vi "Extract Doubles.vi"(1 "String":string="53k, 42M, 37u", 2 "Eng Units?":bool) -> (0 "Data":dbl[](array[numeric]) format="%.5e")   [LabVIEW 2018]
doc: "Finds all numbers in the given string and puts them into an array as double-precision numbers. All of the following formats are recognized:\n123 1.23 1.23e2 1.23E2\nNo spaces or other characters may appear within the number, but any characters may appear before or after the number.\nThe engineering units convers suffixes k,m,u as 1000, 0.001 and 1e-6 multipliers. Case of the units is not important which means that \"M\" is the same as \"m\" and denotes a 0.001 multiplier.\nModified from examples which did not work, by\nScott Hannahs, <sth@magnet.fsu.edu> NHMFL-FSU, May 2003\nAuthor: Scott Hannahs <sth@magnet.fsu.edu>\nCopyright 2018 Florida State University, All rights reserved."
panel:
  # "This VI takes a string containing multiple numbers and\nextracts those numbers into an array.  See the Get Info\ndialog box for more information."
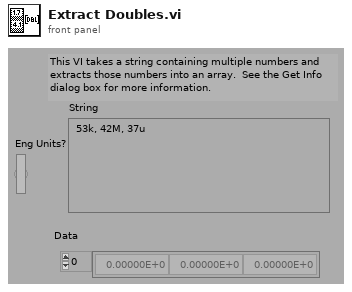
[diagram p1: front panel]
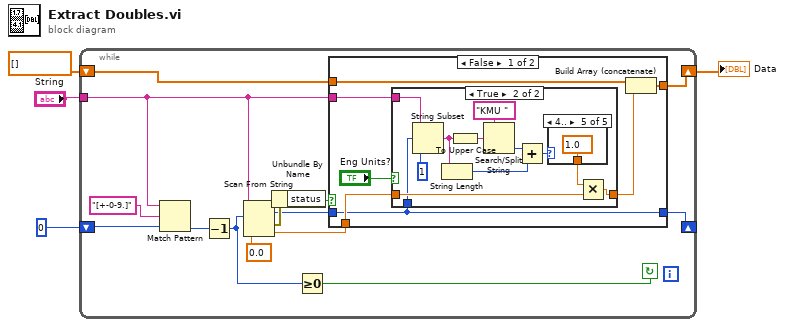
[diagram p0: block diagram]
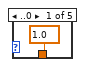
[diagram p3: hidden frame]
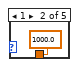
[diagram p4: hidden frame]
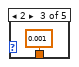
[diagram p5: hidden frame]
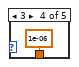
[diagram p6: hidden frame]
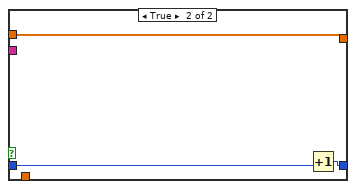
[diagram p7: hidden frame]
diagram:
  n1 = while {
    shift-left: dbl[] [] ("Double Precision Array") -> [w8]
    shift-right: [w7] -> w2
    tunnel: "String" -> [w5]
    shift-left: 0 -> [w17]
    shift-right: [w11] -> _
    stop <- w9 continue-if-true
    n2 = Match Pattern(string=w5, regular expression="[+-0-9.]", offset (0)=w17) -> (offset past match=w16:i32)  [unwired: 3 out]
    n3 = Decrement(x=w16) -> (x-1=w15:i32)
    n4 = Scan From String(input string=w5, initial scan location=w15, default 1=0.0) -> (offset past scan=w10:u32, error out=w13:errorcluster, output 1=w6:dbl)  [unwired: 2 in, 1 out]
    n5 = Unbundle By Name(w13) -> ("status"=w12:bool)
    n6 = Greater Or Equal To 0?(x=w15) -> (x >= 0?=w9:bool)
    n7 = case shown="False" w12 {
      tunnel: [w19 w46] -> w11
      tunnel: w10 -> [w19 w45]
      tunnel: w8 -> [w25 w44]
      tunnel: [w24 w44] -> w7
      tunnel: w6 -> [w22 _]
      tunnel: w5 -> [w20 _]
      frame False {
        n8 = case shown="True" "Eng Units?" {
          tunnel: [w26 w33] -> w21
          tunnel: w22 -> [w26 w34]
          tunnel: w20 -> [_ w36]
          tunnel: w19 -> [_ w32]
          frame False {
          }
          frame True {
            n9 = String Subset(string=w36, offset (0)=w32, length (rest)=1 ("length")) -> (substring=w30:string)
            n10 = String Length(string=w30) -> (length=w27:i32)
            n11 = To Upper Case(1:w30) -> (0:w31:string)
            n12 = Search/Split String(string="KMU ", search string/char (-)=w31) -> (offset of match=w28:i32)  [unwired: 1 in, 2 out]
            n13 = Add(x=w28, y=w27) -> (x+y=w29:i32)
            n14 = case shown="4.." w29 {
              tunnel: [1.0 ("y") 1000.0 ("y") 0.001 ("y") 1e-06 ("y") 1.0 ("y")] -> w35
              frame ..0 {
              }
              frame 1 {
              }
              frame 2 {
              }
              frame 3 {
              }
              frame 4.. {
              }
            }
            n15 = Multiply(x=w35, y=w34) -> (x*y=w33:dbl)
          }
        }
        n16 = Build Array (concatenate)(w25, w21) -> (w24:dbl[])
      }
      frame True {
        n17 = Increment(x=w45) -> (x+1=w46:u32)
      }
    }
  }
  "Data" <- w2
